vi "CLD 12 Sequencer State Machine solution.vi"() -> ()   [LabVIEW 2009]
doc: "CLD 12: Sequenziert boolesche Werte in der Reihenfolge, in der die Werte aus der Datei geladen werden."
uses:
  CLD 12 Sequencer Enum.ctl
  CLD 12 Data Cluster.ctl
  CLD12 Timer Enum.ctl
panel:
  out "Aktuelle Zielzeit":dbl
  in  "Fehler (Eingang, kein Fehler)":errorcluster
  out "Fehler (Ausgang)":errorcluster
  in  "Stopp-Schaltfläche":bool
  out "Verstrichene Zeit":dbl
  out "Schalter 3":bool
  out "Schalter 2":bool
  out "Schalter 1":bool
  in  "Start":bool
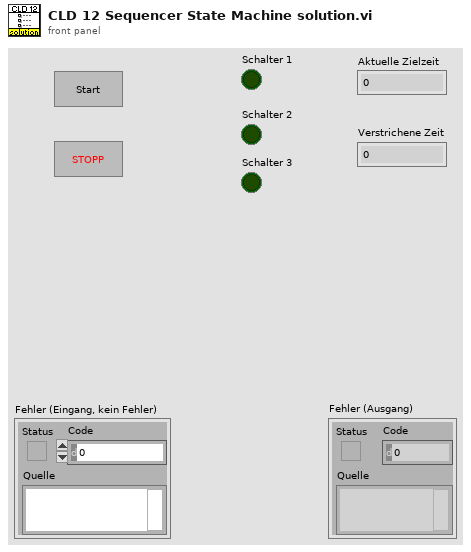
[diagram p1: front panel]
types:
  T1 = typedef "CLD 12 Data Cluster.ctl" = cluster{"Befehl":T2, "Zeitwert":dbl, "Boolesch":bool, "Boolesch 2":bool, "Boolesch 3":bool}
  T2 = typedef "CLD 12 Sequencer Enum.ctl" = enum16{"Initialisieren", "SetTime", "RunState1", "Runstate2", "Ruhezustand", "Starten"}
  T3 = typedef "CLD12 Timer Enum.ctl" = enum16{"Timer starten", "Zeit lesen", "Anhalten", "Fortsetzen", "Timer zurücksetzen"}
  T4 = cluster{"Status":bool, "Code":i32, "Quelle":string}
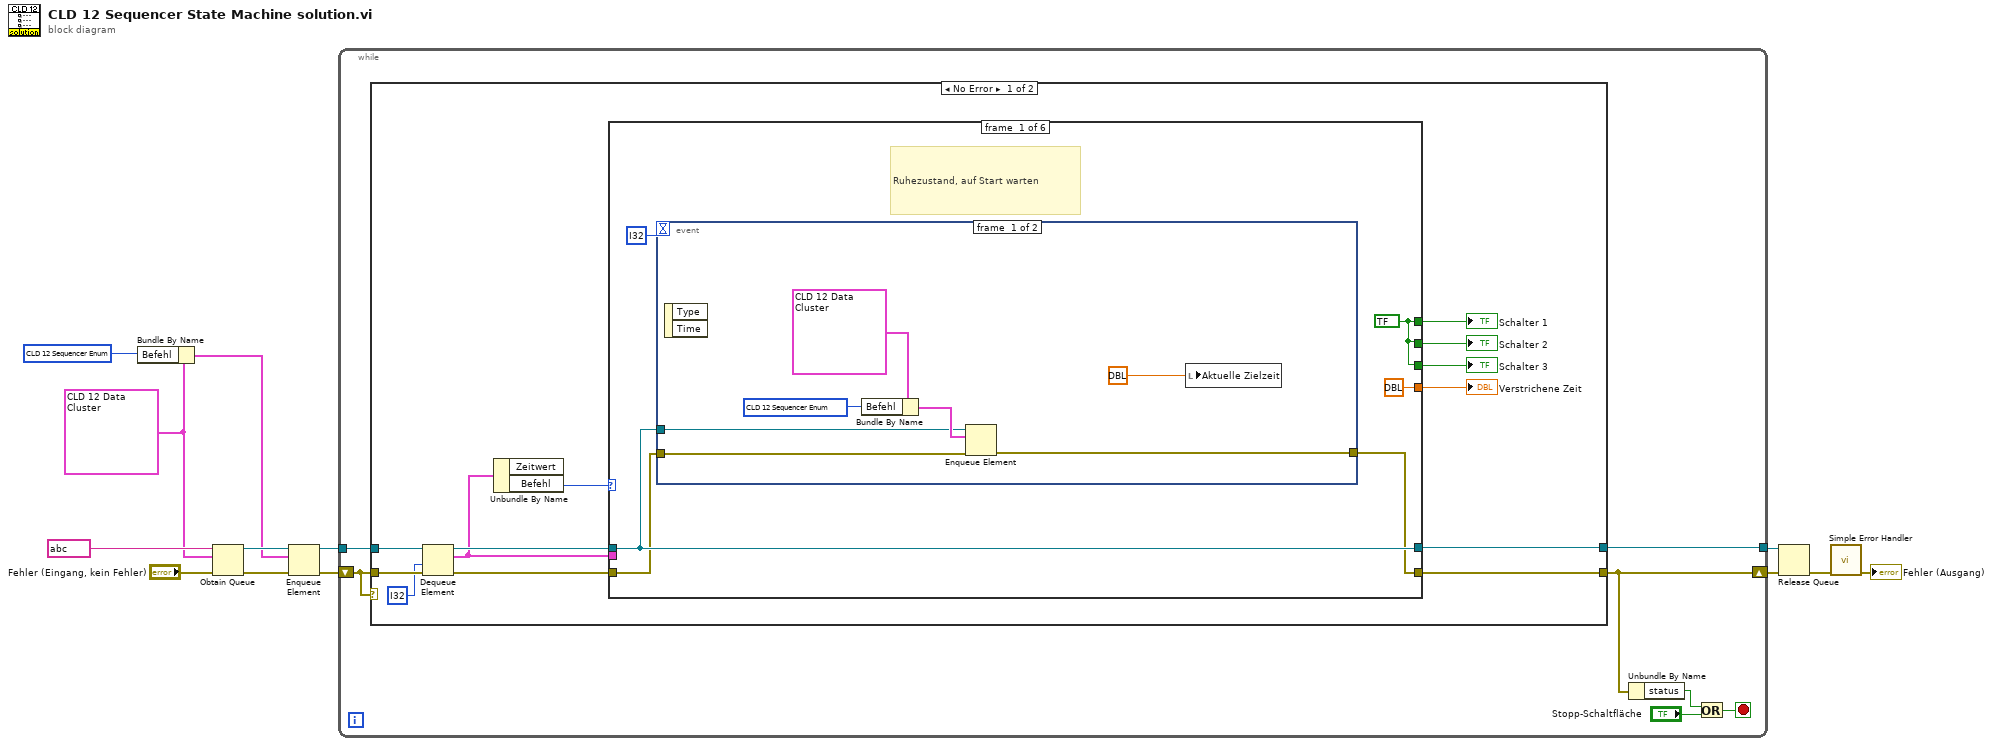
[diagram p0: block diagram]
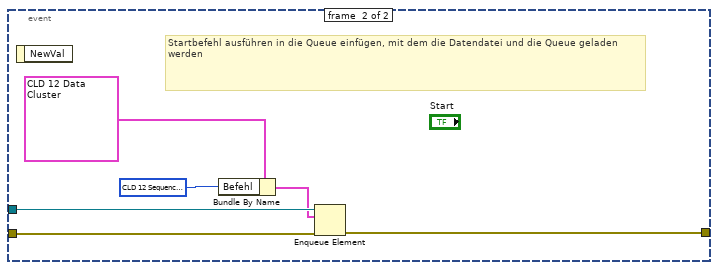
[diagram p2: hidden frame]
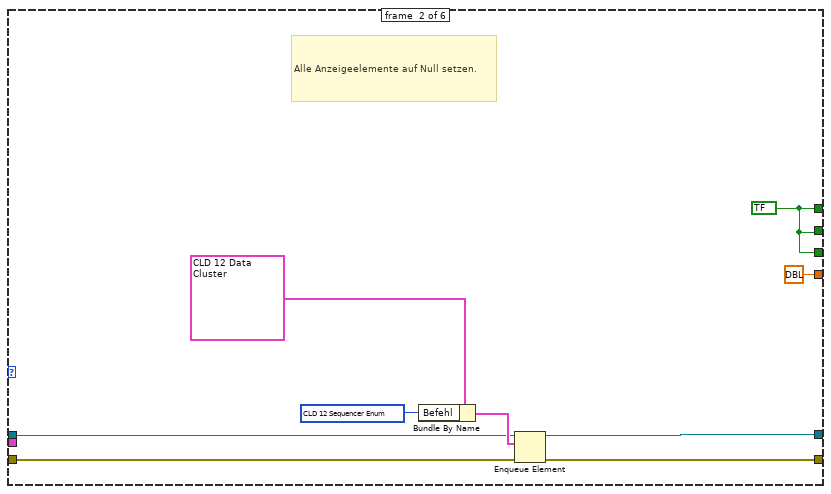
[diagram p3: hidden frame]
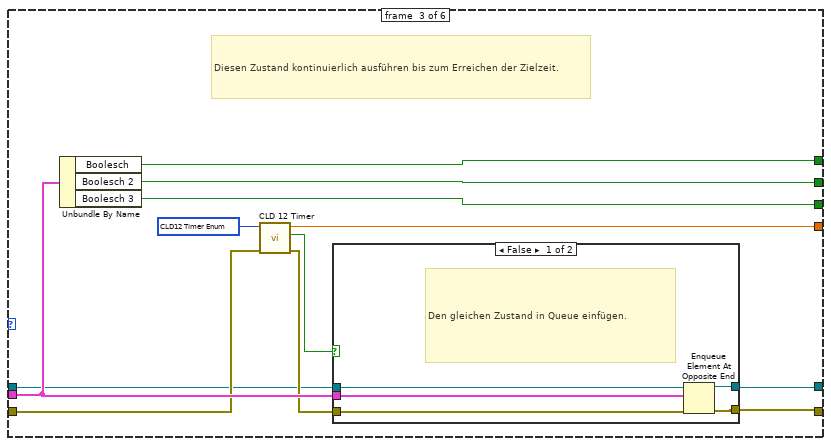
[diagram p4: hidden frame]
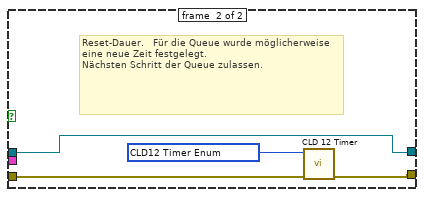
[diagram p5: hidden frame]
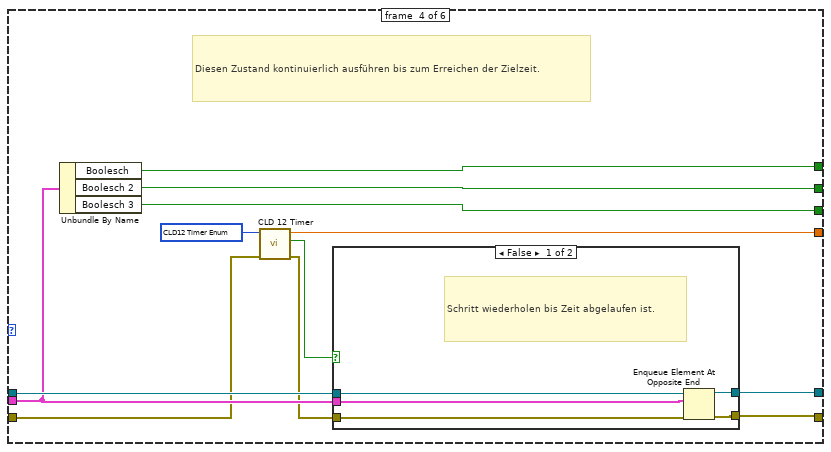
[diagram p6: hidden frame]
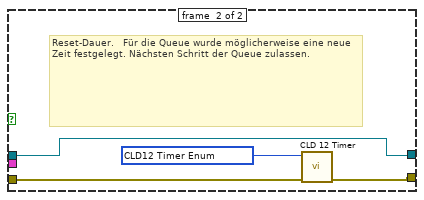
[diagram p7: hidden frame]
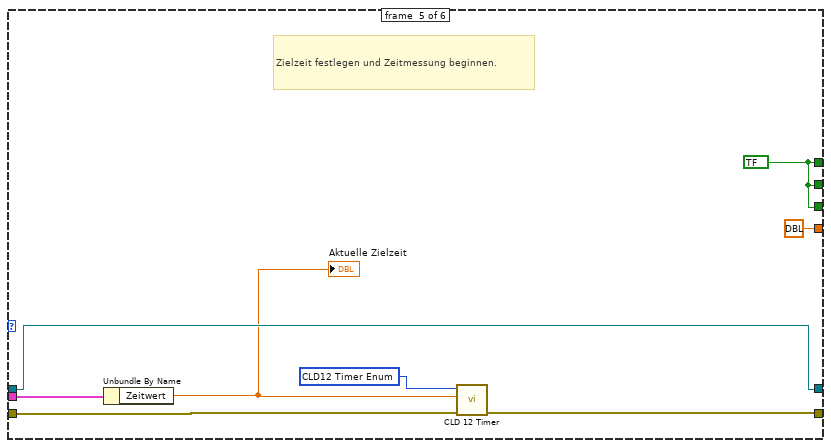
[diagram p8: hidden frame]
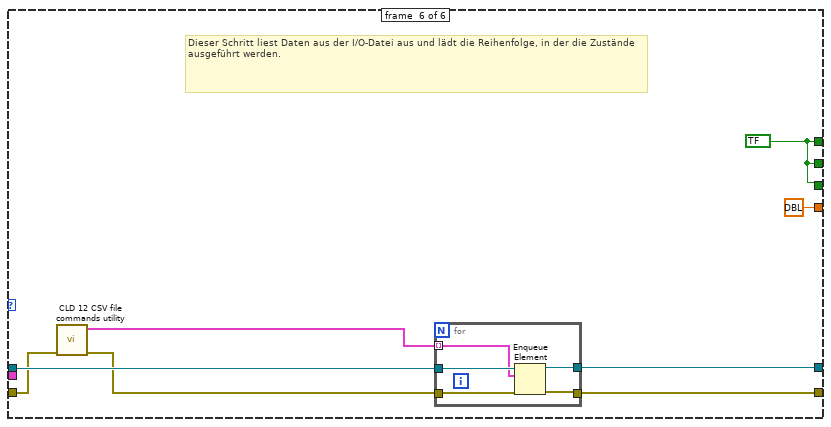
[diagram p9: hidden frame]
diagram:
  w8 = T1 ? ("CLD 12 - Daten-Cluster")
  n1 = Bundle By Name(cluster=w8, "Befehl"=T2 ? ("CLD 12 - Sequenzierelement")) -> (w7:T1)
  n2 = Obtain Queue(name (unnamed)=string ? ("Name (unbenannt)"), element data type=w8, error in (no error)="Fehler (Eingang, kein Fehler)") -> (queue out=w11:refnum<queue>, error out=w13:errorcluster)  [unwired: 2 in, 1 out]
  n3 = Enqueue Element(queue=w11, element=w7, error in (no error)=w13) -> (queue out=w10:refnum<queue>, error out=w12:errorcluster)  [unwired: 1 in, 1 out]
  n4 = while {
    tunnel: w10 -> [w20]
    shift-right: [w16] -> w5
    shift-left: w12 -> [w18]
    tunnel: [w15] -> w4
    stop <- w17 stop-if-true
    n5 = case shown="No Error" w18 {
      tunnel: [w33 w126] -> w16
      tunnel: w20 -> [w32 w125]
      tunnel: w18 -> [w30 w126]
      tunnel: [w22 w125] -> w15
      frame #0 {
        n6 = Dequeue Element(queue=w32, timeout in ms (-1)=i32 ? ("Timeout in ms (-1)"), error in (no error)=w30) -> (queue out=w31:refnum<queue>, element=w27:T1, error out=w29:errorcluster)  [unwired: 1 out]
        n7 = Unbundle By Name(w27) -> ("Befehl"=w28:T2)  [unwired: 1 out]
        n8 = case shown="\"SetTime\"" w28 {
          tunnel: [w36 w57 w67 w87 w110 w118] -> w33
          tunnel: w29 -> [w37 w58 w66 w86 w111 w116]
          tunnel: w31 -> [w39 w54 w64 w94 w106 w119]
          tunnel: w27 -> [_ _ w68 w88 w109 _]
          tunnel: [w35 w56 w73 w93 w108 w114] -> w26
          tunnel: [w35 w56 w72 w92 w108 w114] -> w25
          tunnel: [w35 w56 w71 w91 w108 w114] -> w24
          tunnel: [dbl ? ("Verstrichene Zeit (s,ss)") dbl ? ("Verstrichene Zeit (s,ss)") w70 w90 dbl ? ("Verstrichene Zeit (s,ss)") dbl ? ("Verstrichene Zeit (s,ss)")] -> w23
          tunnel: [w39 w53 w63 w84 w106 w112] -> w22
          frame #0 {
            w35 = bool ? ("Boolesch 1")
            # "Ruhezustand, auf Start warten"
            n9 = event shown="[1] \"Start\": Value Change" {
              selector: _ -> [_ _]
              dyn-events: _ -> [_ _]
              timeout: i32 ? -> [_ _]
              tunnel: w37 -> [w42 w52]
              tunnel: w39 -> [w43 w51]
              tunnel: [w41 w47] -> w36
              event #0 {
                n10 = event-data() -> ()  [unwired: 1 in, 2 out]
                n11 = Bundle By Name(cluster=T1 ? ("CLD 12 - Daten-Cluster"), "Befehl"=T2 ? ("CLD 12 - Sequenzierelement")) -> (w44:T1)
                n12 = Enqueue Element(queue=w43, element=w44, error in (no error)=w42) -> (error out=w41:errorcluster)  [unwired: 1 in, 2 out]
                n13 = local write "Aktuelle Zielzeit"(dbl ? ("Aktuelle Zeit")) -> ()
              }
              event #1 {
                # "Startbefehl ausführen in die Queue einfügen, mit dem die Datendatei und die Queue geladen werden"
                n14 = event-data() -> ()  [unwired: 1 in, 1 out]
                n15 = Bundle By Name(cluster=T1 ? ("CLD 12 - Daten-Cluster"), "Befehl"=T2 ? ("CLD 12 - Sequenzierelement")) -> (w48:T1)
                n16 = Enqueue Element(queue=w51, element=w48, error in (no error)=w52) -> (error out=w47:errorcluster)  [unwired: 1 in, 2 out]
              }
            }
          }
          frame #1 {
            w56 = bool ? ("Boolesch 1")
            # "Alle Anzeigeelemente auf Null setzen."
            n17 = Bundle By Name(cluster=T1 ? ("CLD 12 - Daten-Cluster"), "Befehl"=T2 ? ("CLD 12 - Sequenzierelement")) -> (w59:T1)
            n18 = Enqueue Element(queue=w54, element=w59, error in (no error)=w58) -> (queue out=w53:refnum<queue>, error out=w57:errorcluster)  [unwired: 1 in, 1 out]
          }
          frame #2 {
            # "Diesen Zustand kontinuierlich ausführen bis zum Erreichen der Zielzeit."
            n19 = Unbundle By Name(w68) -> ("Boolesch"=w73:bool, "Boolesch 2"=w72:bool, "Boolesch 3"=w71:bool)
            n20 = call "CLD 12 Timer.vi"("Fehler (Eingang)"=w66, "CLD 12 - Timer-Enum"=T3 ? ("CLD 12 - Zeit-Enum")) -> ("Fehler (Ausgang)"=w65:T4, "Ist Zeit verstrichen?"=w69:bool, "Verstrichene Zeit (s,ms)"=w70:dbl)  [unwired: 7 in]
            n21 = case shown="False" w69 {
              tunnel: w64 -> [w78 w79]
              tunnel: w68 -> [w77 _]
              tunnel: w65 -> [w76 w82]
              tunnel: [w75 w81] -> w67
              tunnel: [w74 w79] -> w63
              frame #0 {
                # "Den gleichen Zustand in Queue einfügen."
                n22 = Enqueue Element At Opposite End(queue=w78, element=w77, error in (no error)=w76) -> (queue out=w74:refnum<queue>, error out=w75:errorcluster)  [unwired: 1 in, 1 out]
              }
              frame #1 {
                # "Reset-Dauer.   Für die Queue wurde möglicherweise eine neue Zeit festgelegt.\nNächsten Schritt der Queue zulassen."
                n23 = call "CLD 12 Timer.vi"("Fehler (Eingang)"=w82, "CLD 12 - Timer-Enum"=T3 ? ("CLD 12 - Enum")) -> ("Fehler (Ausgang)"=w81:T4)  [unwired: 7 in, 2 out]
              }
            }
          }
          frame #3 {
            # "Diesen Zustand kontinuierlich ausführen bis zum Erreichen der Zielzeit."
            n24 = Unbundle By Name(w88) -> ("Boolesch"=w93:bool, "Boolesch 2"=w92:bool, "Boolesch 3"=w91:bool)
            n25 = call "CLD 12 Timer.vi"("Fehler (Eingang)"=w86, "CLD 12 - Timer-Enum"=T3 ? ("CLD 12 - Zeit-Enum")) -> ("Fehler (Ausgang)"=w85:T4, "Ist Zeit verstrichen?"=w89:bool, "Verstrichene Zeit (s,ms)"=w90:dbl)  [unwired: 7 in]
            n26 = case shown="False" w89 {
              tunnel: w94 -> [w99 w100]
              tunnel: w88 -> [w98 _]
              tunnel: w85 -> [w97 w103]
              tunnel: [w96 w102] -> w87
              tunnel: [w95 w100] -> w84
              frame #0 {
                # "Schritt wiederholen bis Zeit abgelaufen ist."
                n27 = Enqueue Element At Opposite End(queue=w99, element=w98, error in (no error)=w97) -> (queue out=w95:refnum<queue>, error out=w96:errorcluster)  [unwired: 1 in, 1 out]
              }
              frame #1 {
                # "Reset-Dauer.   Für die Queue wurde möglicherweise eine neue Zeit festgelegt. Nächsten Schritt der Queue zulassen."
                n28 = call "CLD 12 Timer.vi"("Fehler (Eingang)"=w103, "CLD 12 - Timer-Enum"=T3 ? ("CLD 12 - Enum")) -> ("Fehler (Ausgang)"=w102:T4)  [unwired: 7 in, 2 out]
              }
            }
          }
          frame #4 {
            w108 = bool ? ("Boolesch 1")
            # "Zielzeit festlegen und Zeitmessung beginnen."
            n29 = Unbundle By Name(w109) -> ("Zeitwert"=w104:dbl)
            "Aktuelle Zielzeit" <- w104
            n30 = call "CLD 12 Timer.vi"("Fehler (Eingang)"=w111, "Zielzeit (s)"=w104, "CLD 12 - Timer-Enum"=T3 ? ("CLD 12 - Zeit-Enum")) -> ("Fehler (Ausgang)"=w110:T4)  [unwired: 6 in, 2 out]
          }
          frame #5 {
            w114 = bool ? ("Boolesch 1")
            # "Dieser Schritt liest Daten aus der I/O-Datei aus und lädt die Reihenfolge, in der die Zustände ausgeführt werden."
            n31 = call "CLD 12 CSV file commands utility.vi"("Fehler (Eingang)"=w116) -> ("Fehler (Ausgang)"=w115:T4, "Befehls-Ausgangs-Array"=w117:T1[])  [unwired: 9 in]
            n32 = for {
              tunnel: w119 -> [w124]
              tunnel: [w121] -> w118
              tunnel: w115 -> [w123]
              tunnel: w117 -> [w122] mode=indexing
              tunnel: [w120] -> w112
              n33 = Enqueue Element(queue=w124, element=w122, error in (no error)=w123) -> (queue out=w120:refnum<queue>, error out=w121:errorcluster)  [unwired: 1 in, 1 out]
            }
          }
        }
        "Verstrichene Zeit" <- w23
        "Schalter 1" <- w26
        "Schalter 2" <- w25
        "Schalter 3" <- w24
      }
      frame #1 {
      }
    }
    n34 = Unbundle By Name(w16) -> ("status"=w14:bool)
    n35 = Or(x=w14, y="Stopp-Schaltfläche") -> (x .or. y?=w17:bool)
  }
  n36 = Release Queue(queue=w4, error in (no error)=w5) -> (error out=w3:errorcluster)  [unwired: 1 in, 2 out]
  n37 = call <vilib>:"Simple Error Handler.vi"("error in (no error)"=w3) -> ("error out"=→"Fehler (Ausgang)":errorcluster)  [unwired: 4 in, 4 out]
